vi "GUI_Single Button Pump.vi"() -> ()   [LabVIEW 2011] (continued)
                            n349 = call "MID-VAC Timer.vi"("TO sec (Start timer)"=30.0, "Action"=timerAction_typdef."Start Timer") -> ()  [unwired: 9 in, 1 out]
                            n350 = Concatenate Strings("Main: HPD Sanity Check>>", w961) -> (w960:string)
                          }
                          frame "Continue to Wait" {
                            # "Continue to wait. Reset Timer"
                            n351 = call "MID-VAC Timer.vi"("TO sec (Start timer)"=30.0, "Action"=timerAction_typdef."Start Timer") -> ()  [unwired: 9 in, 1 out]
                            n352 = Concatenate Strings("Main: HPD Sanity Check>>", w965) -> (w966:string)
                          }
                          frame "Exit" {
                          }
                        }
                      }
                      frame True {
                        n353 = Concatenate Strings("Main: HPD Sanity Check>>", w972) -> (w971:string)
                      }
                    }
                  }
                }
                n354 = call "MID-VAC Timer.vi"("Action"=timerAction_typdef."Timer Running") -> ("TO"=w925:bool)  [unwired: 10 in]
                n355 = And(x=w920, y=w925) -> (x .and. y?=w924:bool)
                n356 = Concatenate Strings(w916, " Valve is NOT Closed. Perform corrective action.\nClick on continue to wait for some more time.\nClick Exit to abort GPM" ("message")) -> (w917:string)
                n357 = call "Generate TO event.vi"("Boolean"=w924, "message"=w917, "User Event in"=w927) -> ()  [unwired: 9 in]
              }
            }
          }
        }
        n358 = call <vilib>:"Add State(s) to Queue__jki_lib_state_machine.vi"("State(s) in Front (\"\")"=w895, "State(s) in (\"\")"=w890) -> ("States Out"=w900:string)  [unwired: 13 in]
      }
      frame "Main: HPBD Sanity Check" {
        # "Check if gate valve between COMP and M123 is Open"
        n359 = Unbundle By Name(w976) -> ("Chamber Selection.M123"=w979:bool, "Chamber Selection.HPBD"=w980:bool)
        n360 = case shown="True" w980 {
          tunnel: w985 -> [w989 w998]
          tunnel: w984 -> [_ w997]
          tunnel: [w989 w996] -> w983
          tunnel: w982 -> [_ w995]
          tunnel: ["" w994] -> w981
          tunnel: w976 -> [w987 w993]
          tunnel: w979 -> [_ w991]
          tunnel: w978 -> [_ w992]
          tunnel: [w987 w990] -> w975
          frame False {
          }
          frame True {
            # "Check Conditions"
            n361 = case shown="\"False\", Default" w992 {
              selector: w992 -> [_ w1011]
              tunnel: w998 -> [w1003 w1013]
              tunnel: w997 -> [_ _]
              tunnel: [w1003 w1004] -> w996
              tunnel: w995 -> [_ _]
              tunnel: [w1001 ""] -> w994
              tunnel: w993 -> [w999 w1010]
              tunnel: w991 -> [w1000 _]
              tunnel: [w999 w1009] -> w990
              frame "False", Default {
                w1002 = "Main: HPBD Sanity Check>>M123-HPBD"
                # "COMP SELECTED?"
                n362 = Select(t=w1002, s=w1000, f=w1002) -> (s? t:f=w1001:string)
              }
              frame "M123-HPBD" {
                # "Event TAG"
                n363 = case shown="\"M123-HPBD\"" w1011 {
                  tunnel: [w1015 w1016] -> w1014
                  frame "False", Default {
                    w1015 = T32[] [enum."No Action"] items=["No Action", "Is EC GPM Mode ON?", "Is EC GPM Mode Off?", "Is EC GVM Mode ON?", "Is EC GVM Off?", "Is  EC GPM or GVM Mode ON?", "Is LB GPM Mode ON?", "Is LB GPM Mode Off?", "Is LB GVM Mode ON?", "Is LB GVM Mode Off?", "Is  LB GPM or GVM Mode ON?", "Is M123 Turbo Gate Valve Opened? ", "Is M123 Turbo Gate Valve Closed?", "Is OAP Turbo Gate Valve Opened?", "Is OAP Turbo Gate Valve Closed?", "Is BTLTurbo Gate Valve Opened?", "Is BTL Turbo Gate Valve Closed?", "Is TARGET Turbo Gate Valve 1Opened?", "Is TARGET1 Turbo Gate Valve Closed?", "Is TARGET Turbo Gate Valve 2 Opened?", "Is TAREGT2 Turbo Gate Valve Closed?", "Is BTL2 Turbo Gate Valve Opened?", "Is BTL2 Turbo Gate Valve Closed?", "Is HPD Turbo Gate Valve Opened?", "Is HPD Turbo Gate Valve Closed?", "Is COMP to M123 gate Valve Opened?", "Is COMP to M123 Valve Closed?", "Is HPBD Gate Valve Opened?", "Is HPBD Gate Valve Closed?", "Is M123 to OAP gate valve opened?", "Is M123 to OAP gate valve closed?", "Is OAP to BLT gate valve opened?", "Is OAP to BTL Gate Valve Closed?", "Is BLT to TARGET gate valve opened?", "Is BTL to TARGET Gate Valve Closed?", "Is TARGET to BLT2 gate valve opened?", "Is TARGET to BTL2 Gate Valve Closed?", "Is BLT2 to HPD gate valve opened?", "Is BTL2 to HPD Gate Valve Closed?", "Is COMP at Atmospheric Pressure?", "Is M123 at Atmospheric Pressure?", "Is BeamDump at Atmospheric Pressure?", "Is OAP at Atmospheric Pressure?", "Is BLT at Atmospheric Pressure", "Is TARGET at Atmospheric Pressure?", "Is BLT2 at Atmospheric Pressure?", "Is HPD at Atmospheric Pressure?", "Is the EC Roughing Pump ON?", "Is the EC Roughing Pump OFF?", "Does the EC Roughing Pump have a fault?", "Is the LB Roughing Pump ON?", "Is the LB Roughing Pump Off?", "Does the LB Roughing Pump have a fault?", "Is the EC Backing Pump ON?", "Is the EC Backing Pump OFF?", "Is the LB Backing Pump ON?", "Is the LB Backing Pump OFF?", "Does the EC Backing Pump have a fault?", "Does the LB Backing Pump have a fault?", "Is the EC Backing Pipe at Atmospheric Pressure", "Is the LB Backing Pipe at Atmospheric Pressure", "Is the EC Backing Manifold at Atmospheric Pressure", "s the LB Backing Manifold at Atmospheric Pressure?", "Is the EC Roughing Pipe at Atmospheric Pressure", "Is the LB Roughing Pipe at Atmospheric Pressure?", "Is the EC Roughing Manifold at Atmospheric Pressure", "Is the LB Roughing Manifold at Atmospheric Pressure", "Is LB Backing Manifold Valve Opened?", "Is EC Backing Manifold Valve Opened?", "Is LB Roughing Manifold Valve Opened?", "Is EC Roughing Manifold Valve Opened?", "Is COMP Roughing Valve Opened?", "Is M123 Roughing Valve Opened?", "Is M123 Roughing Valve Closed?", "Is OAP Roughing Valve Opened?", "Is OAP Roughing Valve Closed?", "Is HPBD Roughing Valve Opened?", "Is HPBD Roughing Valve Closed?", "Is BTL Roughing Valve Opened?", "Is BTL Roughing Valve Closed?", "Is TARGET Roughing Valve Opened?", "Is TARGET Roughing Valve Closed?", "Is BTL2 Roughing Valve Opened?", "Is BTL2 Roughing Valve Closed?", "Is HPD Roughing Valve Opened?", "Is HPD Roughing Valve Closed?", "Is COMP Turbo Backing Valve Opened?", "Is M123 Turbo Backing Valve Opened", "Is HPBD Turbo Backing Valve Opened?", "Is OAP Turbo Backing Valve Opened?", "Is BTL Turbo Backing Valve Opened?", "Is TARGET1 Turbo Backing Valve Opened?", "Is TARGET2 Turbo Backing Valve Opened?", "Is BTL2 Turbo Backing Valve Opened?", "Is HPD Turbo Backing Valve Opened?", "Is M123 Backing at MID-VAC?", "Is OAP Backing at MID-VAC?", "Is TARGET1 Backing at MID-VAC?", "Is TARGET2 Backing at MID-VAC?", "Is BTL Backing at MID-VAC?", "Is BTL2 Backing at MID-VAC?", "Is HPD Backing at MID-VAC?", "Is M123 Turbo in Normal Operation", "Is COMP Turbo in Normal Operation", "Is OAP Turbo in Normal Operation", "Is BTL Turbo in Normal Operation", "Is TARGET1 Turbo in Normal Operation", "Is TARGET2 Turbo in Normal Operation", "Is BTL2 Turbo in Normal Operation", "Is HPD Turbo in Normal Operation", "Is M123 at MID-VAC?", "Is OAP at MID-VAC?", "Is COMP at MID-VAC?", "Is BTL at MID-VAC?", "Is TARGET at MID-VAC?", "Is BTL2 at MID-VAC?", "Is HPD at MID-VAC?"]
                  }
                  frame "M123-HPBD" {
                    w1016 = T32[] [enum."Is HPBD Gate Valve Closed?"] items=["No Action", "Is EC GPM Mode ON?", "Is EC GPM Mode Off?", "Is EC GVM Mode ON?", "Is EC GVM Off?", "Is  EC GPM or GVM Mode ON?", "Is LB GPM Mode ON?", "Is LB GPM Mode Off?", "Is LB GVM Mode ON?", "Is LB GVM Mode Off?", "Is  LB GPM or GVM Mode ON?", "Is M123 Turbo Gate Valve Opened? ", "Is M123 Turbo Gate Valve Closed?", "Is OAP Turbo Gate Valve Opened?", "Is OAP Turbo Gate Valve Closed?", "Is BTLTurbo Gate Valve Opened?", "Is BTL Turbo Gate Valve Closed?", "Is TARGET Turbo Gate Valve 1Opened?", "Is TARGET1 Turbo Gate Valve Closed?", "Is TARGET Turbo Gate Valve 2 Opened?", "Is TAREGT2 Turbo Gate Valve Closed?", "Is BTL2 Turbo Gate Valve Opened?", "Is BTL2 Turbo Gate Valve Closed?", "Is HPD Turbo Gate Valve Opened?", "Is HPD Turbo Gate Valve Closed?", "Is COMP to M123 gate Valve Opened?", "Is COMP to M123 Valve Closed?", "Is HPBD Gate Valve Opened?", "Is HPBD Gate Valve Closed?", "Is M123 to OAP gate valve opened?", "Is M123 to OAP gate valve closed?", "Is OAP to BLT gate valve opened?", "Is OAP to BTL Gate Valve Closed?", "Is BLT to TARGET gate valve opened?", "Is BTL to TARGET Gate Valve Closed?", "Is TARGET to BLT2 gate valve opened?", "Is TARGET to BTL2 Gate Valve Closed?", "Is BLT2 to HPD gate valve opened?", "Is BTL2 to HPD Gate Valve Closed?", "Is COMP at Atmospheric Pressure?", "Is M123 at Atmospheric Pressure?", "Is BeamDump at Atmospheric Pressure?", "Is OAP at Atmospheric Pressure?", "Is BLT at Atmospheric Pressure", "Is TARGET at Atmospheric Pressure?", "Is BLT2 at Atmospheric Pressure?", "Is HPD at Atmospheric Pressure?", "Is the EC Roughing Pump ON?", "Is the EC Roughing Pump OFF?", "Does the EC Roughing Pump have a fault?", "Is the LB Roughing Pump ON?", "Is the LB Roughing Pump Off?", "Does the LB Roughing Pump have a fault?", "Is the EC Backing Pump ON?", "Is the EC Backing Pump OFF?", "Is the LB Backing Pump ON?", "Is the LB Backing Pump OFF?", "Does the EC Backing Pump have a fault?", "Does the LB Backing Pump have a fault?", "Is the EC Backing Pipe at Atmospheric Pressure", "Is the LB Backing Pipe at Atmospheric Pressure", "Is the EC Backing Manifold at Atmospheric Pressure", "s the LB Backing Manifold at Atmospheric Pressure?", "Is the EC Roughing Pipe at Atmospheric Pressure", "Is the LB Roughing Pipe at Atmospheric Pressure?", "Is the EC Roughing Manifold at Atmospheric Pressure", "Is the LB Roughing Manifold at Atmospheric Pressure", "Is LB Backing Manifold Valve Opened?", "Is EC Backing Manifold Valve Opened?", "Is LB Roughing Manifold Valve Opened?", "Is EC Roughing Manifold Valve Opened?", "Is COMP Roughing Valve Opened?", "Is M123 Roughing Valve Opened?", "Is M123 Roughing Valve Closed?", "Is OAP Roughing Valve Opened?", "Is OAP Roughing Valve Closed?", "Is HPBD Roughing Valve Opened?", "Is HPBD Roughing Valve Closed?", "Is BTL Roughing Valve Opened?", "Is BTL Roughing Valve Closed?", "Is TARGET Roughing Valve Opened?", "Is TARGET Roughing Valve Closed?", "Is BTL2 Roughing Valve Opened?", "Is BTL2 Roughing Valve Closed?", "Is HPD Roughing Valve Opened?", "Is HPD Roughing Valve Closed?", "Is COMP Turbo Backing Valve Opened?", "Is M123 Turbo Backing Valve Opened", "Is HPBD Turbo Backing Valve Opened?", "Is OAP Turbo Backing Valve Opened?", "Is BTL Turbo Backing Valve Opened?", "Is TARGET1 Turbo Backing Valve Opened?", "Is TARGET2 Turbo Backing Valve Opened?", "Is BTL2 Turbo Backing Valve Opened?", "Is HPD Turbo Backing Valve Opened?", "Is M123 Backing at MID-VAC?", "Is OAP Backing at MID-VAC?", "Is TARGET1 Backing at MID-VAC?", "Is TARGET2 Backing at MID-VAC?", "Is BTL Backing at MID-VAC?", "Is BTL2 Backing at MID-VAC?", "Is HPD Backing at MID-VAC?", "Is M123 Turbo in Normal Operation", "Is COMP Turbo in Normal Operation", "Is OAP Turbo in Normal Operation", "Is BTL Turbo in Normal Operation", "Is TARGET1 Turbo in Normal Operation", "Is TARGET2 Turbo in Normal Operation", "Is BTL2 Turbo in Normal Operation", "Is HPD Turbo in Normal Operation", "Is M123 at MID-VAC?", "Is OAP at MID-VAC?", "Is COMP at MID-VAC?", "Is BTL at MID-VAC?", "Is TARGET at MID-VAC?", "Is BTL2 at MID-VAC?", "Is HPD at MID-VAC?"]
                  }
                }
                n364 = call "GetAction.vi"("Check Condition"=Error_codes."999-No Event" ("Error Codes"), "Query Array"=w1014, "error in (no error)"=w1013) -> ("Results Array"=w1007:bool[], "error out"=w1004:errorcluster)  [unwired: 7 in, 4 out]
                n365 = Index Array(array=w1007, index=0) -> (element=w1005:bool)
                n366 = Bundle By Name(cluster=w1010, "Isolate HPBD"=w1005) -> (w1009:T20)
              }
            }
          }
        }
        n367 = call <vilib>:"Add State(s) to Queue__jki_lib_state_machine.vi"("State(s) in Front (\"\")"=w981, "State(s) in (\"\")"=w977) -> ("States Out"=w986:string)  [unwired: 13 in]
      }
      frame "Main: Check COMP gate valve" {
        w1028 = Error_codes."003-Chamber Gate Valve Status" ("Error Codes")
        w1034 = T32[] [enum."Is COMP to M123 Valve Closed?"] items=["No Action", "Is EC GPM Mode ON?", "Is EC GPM Mode Off?", "Is EC GVM Mode ON?", "Is EC GVM Off?", "Is  EC GPM or GVM Mode ON?", "Is LB GPM Mode ON?", "Is LB GPM Mode Off?", "Is LB GVM Mode ON?", "Is LB GVM Mode Off?", "Is  LB GPM or GVM Mode ON?", "Is M123 Turbo Gate Valve Opened? ", "Is M123 Turbo Gate Valve Closed?", "Is OAP Turbo Gate Valve Opened?", "Is OAP Turbo Gate Valve Closed?", "Is BTLTurbo Gate Valve Opened?", "Is BTL Turbo Gate Valve Closed?", "Is TARGET Turbo Gate Valve 1Opened?", "Is TARGET1 Turbo Gate Valve Closed?", "Is TARGET Turbo Gate Valve 2 Opened?", "Is TAREGT2 Turbo Gate Valve Closed?", "Is BTL2 Turbo Gate Valve Opened?", "Is BTL2 Turbo Gate Valve Closed?", "Is HPD Turbo Gate Valve Opened?", "Is HPD Turbo Gate Valve Closed?", "Is COMP to M123 gate Valve Opened?", "Is COMP to M123 Valve Closed?", "Is HPBD Gate Valve Opened?", "Is HPBD Gate Valve Closed?", "Is M123 to OAP gate valve opened?", "Is M123 to OAP gate valve closed?", "Is OAP to BLT gate valve opened?", "Is OAP to BTL Gate Valve Closed?", "Is BLT to TARGET gate valve opened?", "Is BTL to TARGET Gate Valve Closed?", "Is TARGET to BLT2 gate valve opened?", "Is TARGET to BTL2 Gate Valve Closed?", "Is BLT2 to HPD gate valve opened?", "Is BTL2 to HPD Gate Valve Closed?", "Is COMP at Atmospheric Pressure?", "Is M123 at Atmospheric Pressure?", "Is BeamDump at Atmospheric Pressure?", "Is OAP at Atmospheric Pressure?", "Is BLT at Atmospheric Pressure", "Is TARGET at Atmospheric Pressure?", "Is BLT2 at Atmospheric Pressure?", "Is HPD at Atmospheric Pressure?", "Is the EC Roughing Pump ON?", "Is the EC Roughing Pump OFF?", "Does the EC Roughing Pump have a fault?", "Is the LB Roughing Pump ON?", "Is the LB Roughing Pump Off?", "Does the LB Roughing Pump have a fault?", "Is the EC Backing Pump ON?", "Is the EC Backing Pump OFF?", "Is the LB Backing Pump ON?", "Is the LB Backing Pump OFF?", "Does the EC Backing Pump have a fault?", "Does the LB Backing Pump have a fault?", "Is the EC Backing Pipe at Atmospheric Pressure", "Is the LB Backing Pipe at Atmospheric Pressure", "Is the EC Backing Manifold at Atmospheric Pressure", "s the LB Backing Manifold at Atmospheric Pressure?", "Is the EC Roughing Pipe at Atmospheric Pressure", "Is the LB Roughing Pipe at Atmospheric Pressure?", "Is the EC Roughing Manifold at Atmospheric Pressure", "Is the LB Roughing Manifold at Atmospheric Pressure", "Is LB Backing Manifold Valve Opened?", "Is EC Backing Manifold Valve Opened?", "Is LB Roughing Manifold Valve Opened?", "Is EC Roughing Manifold Valve Opened?", "Is COMP Roughing Valve Opened?", "Is M123 Roughing Valve Opened?", "Is M123 Roughing Valve Closed?", "Is OAP Roughing Valve Opened?", "Is OAP Roughing Valve Closed?", "Is HPBD Roughing Valve Opened?", "Is HPBD Roughing Valve Closed?", "Is BTL Roughing Valve Opened?", "Is BTL Roughing Valve Closed?", "Is TARGET Roughing Valve Opened?", "Is TARGET Roughing Valve Closed?", "Is BTL2 Roughing Valve Opened?", "Is BTL2 Roughing Valve Closed?", "Is HPD Roughing Valve Opened?", "Is HPD Roughing Valve Closed?", "Is COMP Turbo Backing Valve Opened?", "Is M123 Turbo Backing Valve Opened", "Is HPBD Turbo Backing Valve Opened?", "Is OAP Turbo Backing Valve Opened?", "Is BTL Turbo Backing Valve Opened?", "Is TARGET1 Turbo Backing Valve Opened?", "Is TARGET2 Turbo Backing Valve Opened?", "Is BTL2 Turbo Backing Valve Opened?", "Is HPD Turbo Backing Valve Opened?", "Is M123 Backing at MID-VAC?", "Is OAP Backing at MID-VAC?", "Is TARGET1 Backing at MID-VAC?", "Is TARGET2 Backing at MID-VAC?", "Is BTL Backing at MID-VAC?", "Is BTL2 Backing at MID-VAC?", "Is HPD Backing at MID-VAC?", "Is M123 Turbo in Normal Operation", "Is COMP Turbo in Normal Operation", "Is OAP Turbo in Normal Operation", "Is BTL Turbo in Normal Operation", "Is TARGET1 Turbo in Normal Operation", "Is TARGET2 Turbo in Normal Operation", "Is BTL2 Turbo in Normal Operation", "Is HPD Turbo in Normal Operation", "Is M123 at MID-VAC?", "Is OAP at MID-VAC?", "Is COMP at MID-VAC?", "Is BTL at MID-VAC?", "Is TARGET at MID-VAC?", "Is BTL2 at MID-VAC?", "Is HPD at MID-VAC?"]
        # "Event TAG"
        # "Check Conditions"
        # "Check if gate valve between COMP and M123 is Open"
        n368 = call "GetAction.vi"("Check Condition"=w1028, "Query Array"=w1034, "error in (no error)"=w1033) -> ("Status Array Out"=w1029:string[], "Generate Event?"=w1021:bool, "error out"=w1031:errorcluster)  [unwired: 7 in, 3 out]
        n369 = Unbundle By Name(w1025) -> ("VI Refnum"=w1024:refnum<vi>)
        n370 = call "Generate User Event.vi"("Add(t)/Remove(f) Event"=w1021, "error in (no error)"=w1031, "User Event in"=w1032, "Status Array In"=w1029, "Error Codes"=w1028) -> ("error out"=w1030:errorcluster)  [unwired: 5 in, 1 out]
        n371 = Not A Number/Path/Refnum?(number/path/refnum=w1024) -> (NaN/Path/Refnum?=w1023:bool)
        n372 = call "MID-VAC Timer.vi"("Action"=timerAction_typdef."Timer Running") -> ("TO"=w1026:bool)  [unwired: 10 in]
        n373 = case shown="False" w1021 {
          tunnel: ["Main: Check Chamber Pressure" w1050] -> w1022
          tunnel: w1024 -> [w1040 w1049]
          tunnel: w1023 -> [w1041 w1048]
          frame False {
            n374 = case shown="True" w1041 {
              tunnel: w1040 -> [_ w1044]
              frame False {
              }
              frame True {
                n375 = invoke class="VI" method="Abort VI"(reference=w1044) -> (reference out=w1042:refnum<vi>, error out=w1043:errorcluster)  [unwired: 2 in, 1 out]
                n376 = case shown="No Error" w1043 {
                  selector: w1043 -> [w1046 _]
                  tunnel: w1042 -> [w1047 _]
                  frame No Error {
                    n377 = Close Reference(reference=w1047, error in (no error)=w1046) -> (error out=w1045:errorcluster)
                    n378 = invoke on="User Input Panel" class="SubPnl" method="Remove VI"(error in=w1045) -> ()  [unwired: 2 in, 3 out]
                  }
                  frame Error {
                  }
                }
              }
            }
            n379 = call "MID-VAC Timer.vi"("TO sec (Start timer)"=1.0, "Action"=timerAction_typdef."Start Timer") -> ()  [unwired: 9 in, 1 out]
          }
          frame True {
            # "when to is true\nand"
            n380 = case shown="False" w1048 {
              tunnel: w1049 -> [w1054 _]
              tunnel: [w1052 "Main: Check COMP gate valve"] -> w1050
              frame False {
                n381 = call "FindControlByName_VEPS.vi"("control name"="Op Out", "vi refnum"=w1054) -> ("control refnum"=w1056:refnum<vi>)  [unwired: 2 in, 1 out]
                n382 = property class="Ctl"(reference=w1056) -> ("Value"=w1055:variant)  [unwired: 1 in, 2 out]
                n383 = Variant To Data(type=op_typdef."Idle" ("Op Out"), Variant=w1055) -> (data=w1053:T24)  [unwired: 1 in, 1 out]
                n384 = case shown="\"Idle\", Default" w1053 {
                  tunnel: ["Main: Check COMP gate valve" "Main: Check COMP gate valve" "Idle\nMacro: Exit"] -> w1052
                  frame "Idle", Default {
                    n385 = call "MID-VAC Timer.vi"("TO sec (Start timer)"=30.0, "Action"=timerAction_typdef."Start Timer") -> ()  [unwired: 9 in, 1 out]
                  }
                  frame "Continue to Wait" {
                    # "Continue to wait. Reset Timer"
                    n386 = call "MID-VAC Timer.vi"("TO sec (Start timer)"=30.0, "Action"=timerAction_typdef."Start Timer") -> ()  [unwired: 9 in, 1 out]
                  }
                  frame "Exit" {
                  }
                }
              }
              frame True {
              }
            }
          }
        }
        n387 = And(x=w1021, y=w1026) -> (x .and. y?=w1018:bool)
        n388 = call "Generate TO event.vi"("Boolean"=w1018, "message"="The COMP to M123 Valve is NOT Closed.\nClick on continue to wait for some more time.\nClick Exit to abort GPM", "User Event in"=w1020) -> ()  [unwired: 9 in]
        n389 = call <vilib>:"Add State(s) to Queue__jki_lib_state_machine.vi"("State(s) in Front (\"\")"=w1022, "State(s) in (\"\")"=w1036) -> ("States Out"=w1035:string)  [unwired: 13 in]
      }
      frame "Main: Check Chamber Pressure" {
        w1073 = Error_codes."004-Check Chamber Pressures" ("Error Codes")
        w1092 = T32[] [enum."Is HPBD Gate Valve Opened?"] items=["No Action", "Is EC GPM Mode ON?", "Is EC GPM Mode Off?", "Is EC GVM Mode ON?", "Is EC GVM Off?", "Is  EC GPM or GVM Mode ON?", "Is LB GPM Mode ON?", "Is LB GPM Mode Off?", "Is LB GVM Mode ON?", "Is LB GVM Mode Off?", "Is  LB GPM or GVM Mode ON?", "Is M123 Turbo Gate Valve Opened? ", "Is M123 Turbo Gate Valve Closed?", "Is OAP Turbo Gate Valve Opened?", "Is OAP Turbo Gate Valve Closed?", "Is BTLTurbo Gate Valve Opened?", "Is BTL Turbo Gate Valve Closed?", "Is TARGET Turbo Gate Valve 1Opened?", "Is TARGET1 Turbo Gate Valve Closed?", "Is TARGET Turbo Gate Valve 2 Opened?", "Is TAREGT2 Turbo Gate Valve Closed?", "Is BTL2 Turbo Gate Valve Opened?", "Is BTL2 Turbo Gate Valve Closed?", "Is HPD Turbo Gate Valve Opened?", "Is HPD Turbo Gate Valve Closed?", "Is COMP to M123 gate Valve Opened?", "Is COMP to M123 Valve Closed?", "Is HPBD Gate Valve Opened?", "Is HPBD Gate Valve Closed?", "Is M123 to OAP gate valve opened?", "Is M123 to OAP gate valve closed?", "Is OAP to BLT gate valve opened?", "Is OAP to BTL Gate Valve Closed?", "Is BLT to TARGET gate valve opened?", "Is BTL to TARGET Gate Valve Closed?", "Is TARGET to BLT2 gate valve opened?", "Is TARGET to BTL2 Gate Valve Closed?", "Is BLT2 to HPD gate valve opened?", "Is BTL2 to HPD Gate Valve Closed?", "Is COMP at Atmospheric Pressure?", "Is M123 at Atmospheric Pressure?", "Is BeamDump at Atmospheric Pressure?", "Is OAP at Atmospheric Pressure?", "Is BLT at Atmospheric Pressure", "Is TARGET at Atmospheric Pressure?", "Is BLT2 at Atmospheric Pressure?", "Is HPD at Atmospheric Pressure?", "Is the EC Roughing Pump ON?", "Is the EC Roughing Pump OFF?", "Does the EC Roughing Pump have a fault?", "Is the LB Roughing Pump ON?", "Is the LB Roughing Pump Off?", "Does the LB Roughing Pump have a fault?", "Is the EC Backing Pump ON?", "Is the EC Backing Pump OFF?", "Is the LB Backing Pump ON?", "Is the LB Backing Pump OFF?", "Does the EC Backing Pump have a fault?", "Does the LB Backing Pump have a fault?", "Is the EC Backing Pipe at Atmospheric Pressure", "Is the LB Backing Pipe at Atmospheric Pressure", "Is the EC Backing Manifold at Atmospheric Pressure", "s the LB Backing Manifold at Atmospheric Pressure?", "Is the EC Roughing Pipe at Atmospheric Pressure", "Is the LB Roughing Pipe at Atmospheric Pressure?", "Is the EC Roughing Manifold at Atmospheric Pressure", "Is the LB Roughing Manifold at Atmospheric Pressure", "Is LB Backing Manifold Valve Opened?", "Is EC Backing Manifold Valve Opened?", "Is LB Roughing Manifold Valve Opened?", "Is EC Roughing Manifold Valve Opened?", "Is COMP Roughing Valve Opened?", "Is M123 Roughing Valve Opened?", "Is M123 Roughing Valve Closed?", "Is OAP Roughing Valve Opened?", "Is OAP Roughing Valve Closed?", "Is HPBD Roughing Valve Opened?", "Is HPBD Roughing Valve Closed?", "Is BTL Roughing Valve Opened?", "Is BTL Roughing Valve Closed?", "Is TARGET Roughing Valve Opened?", "Is TARGET Roughing Valve Closed?", "Is BTL2 Roughing Valve Opened?", "Is BTL2 Roughing Valve Closed?", "Is HPD Roughing Valve Opened?", "Is HPD Roughing Valve Closed?", "Is COMP Turbo Backing Valve Opened?", "Is M123 Turbo Backing Valve Opened", "Is HPBD Turbo Backing Valve Opened?", "Is OAP Turbo Backing Valve Opened?", "Is BTL Turbo Backing Valve Opened?", "Is TARGET1 Turbo Backing Valve Opened?", "Is TARGET2 Turbo Backing Valve Opened?", "Is BTL2 Turbo Backing Valve Opened?", "Is HPD Turbo Backing Valve Opened?", "Is M123 Backing at MID-VAC?", "Is OAP Backing at MID-VAC?", "Is TARGET1 Backing at MID-VAC?", "Is TARGET2 Backing at MID-VAC?", "Is BTL Backing at MID-VAC?", "Is BTL2 Backing at MID-VAC?", "Is HPD Backing at MID-VAC?", "Is M123 Turbo in Normal Operation", "Is COMP Turbo in Normal Operation", "Is OAP Turbo in Normal Operation", "Is BTL Turbo in Normal Operation", "Is TARGET1 Turbo in Normal Operation", "Is TARGET2 Turbo in Normal Operation", "Is BTL2 Turbo in Normal Operation", "Is HPD Turbo in Normal Operation", "Is M123 at MID-VAC?", "Is OAP at MID-VAC?", "Is COMP at MID-VAC?", "Is BTL at MID-VAC?", "Is TARGET at MID-VAC?", "Is BTL2 at MID-VAC?", "Is HPD at MID-VAC?"]
        # "If F, then all chambers are at ATM"
        # "Check Conditions"
        # "Check if Any Chamber is NOT at ATM?"
        n390 = call "GetAction.vi"("Check Condition"=Error_codes."999-No Event" ("Error Codes"), "Query Array"=w1092, "error in (no error)"=w1091) -> ("Results Array"=w1086:bool[], "error out"=w1089:errorcluster)  [unwired: 7 in, 4 out]
        n391 = Index Array(array=w1086, index=0) -> (element=w1072:bool)
        n392 = Not(x=w1072) -> (.not. x?=w1067:bool)
        n393 = Unbundle By Name(w1071) -> ("Chamber Selection"=w1070:T21)
        n394 = call "Selection ActionBuilder.vi"("Selection Action"=Selection_Action_typdef."Check Chamber Pressure", "Isolate HPBD"=w1067, "Chamber Selection"=w1070) -> ("Action Array Out"=w1068:T32[])  [unwired: 7 in, 1 out]
        n395 = call "GetAction.vi"("Check Condition"=w1073, "Query Array"=w1068, "input cluster"=w1071, "error in (no error)"=w1089) -> ("Status Array Out"=w1075:string[], "Generate Event?"=w1080:bool, "error out"=w1074:errorcluster)  [unwired: 6 in, 3 out]
        n396 = call "Generate User Event.vi"("Add(t)/Remove(f) Event"=w1080, "error in (no error)"=w1074, "User Event in"=w1090, "Status Array In"=w1075, "Error Codes"=w1073) -> ("error out"=w1088:errorcluster)  [unwired: 5 in, 1 out]
        n397 = Unbundle By Name(w1071) -> ("VI Refnum"=w1082:refnum<vi>)
        n398 = Not A Number/Path/Refnum?(number/path/refnum=w1082) -> (NaN/Path/Refnum?=w1081:bool)
        n399 = Bundle By Name(cluster=w1071, "Isolate HPBD"=w1067) -> (w1087:T20)
        n400 = case shown="False" w1080 {
          tunnel: ["Main: Check GPM GVM Mode Status" w1109] -> w1079
          tunnel: w1082 -> [w1099 w1108]
          tunnel: w1081 -> [w1100 w1107]
          frame False {
            n401 = case shown="True" w1100 {
              tunnel: w1099 -> [_ w1103]
              frame False {
              }
              frame True {
                n402 = invoke class="VI" method="Abort VI"(reference=w1103) -> (reference out=w1101:refnum<vi>, error out=w1102:errorcluster)  [unwired: 2 in, 1 out]
                n403 = case shown="No Error" w1102 {
                  selector: w1102 -> [w1105 _]
                  tunnel: w1101 -> [w1106 _]
                  frame No Error {
                    n404 = Close Reference(reference=w1106, error in (no error)=w1105) -> (error out=w1104:errorcluster)
                    n405 = invoke on="User Input Panel" class="SubPnl" method="Remove VI"(error in=w1104) -> ()  [unwired: 2 in, 3 out]
                  }
                  frame Error {
                  }
                }
              }
            }
            n406 = call "MID-VAC Timer.vi"("TO sec (Start timer)"=1.0, "Action"=timerAction_typdef."Start Timer") -> ()  [unwired: 9 in, 1 out]
          }
          frame True {
            # "when to is true\nand"
            n407 = case shown="True" w1107 {
              tunnel: w1108 -> [w1113 _]
              tunnel: [w1111 "Main: Check Chamber Pressure"] -> w1109
              frame False {
                n408 = call "FindControlByName_VEPS.vi"("control name"="Op Out", "vi refnum"=w1113) -> ("control refnum"=w1115:refnum<vi>)  [unwired: 2 in, 1 out]
                n409 = property class="Ctl"(reference=w1115) -> ("Value"=w1114:variant)  [unwired: 1 in, 2 out]
                n410 = Variant To Data(type=op_typdef."Idle" ("Op Out"), Variant=w1114) -> (data=w1112:T24)  [unwired: 1 in, 1 out]
                n411 = case shown="\"Idle\", Default" w1112 {
                  tunnel: ["Main: Check Chamber Pressure" "Main: Check Chamber Pressure" "Idle\nMacro: Exit"] -> w1111
                  frame "Idle", Default {
                    n412 = call "MID-VAC Timer.vi"("TO sec (Start timer)"=30.0, "Action"=timerAction_typdef."Start Timer") -> ()  [unwired: 9 in, 1 out]
                  }
                  frame "Continue to Wait" {
                    # "Continue to wait. Reset Timer"
                    n413 = call "MID-VAC Timer.vi"("TO sec (Start timer)"=30.0, "Action"=timerAction_typdef."Start Timer") -> ()  [unwired: 9 in, 1 out]
                  }
                  frame "Exit" {
                  }
                }
              }
              frame True {
              }
            }
          }
        }
        n414 = call "MID-VAC Timer.vi"("Action"=timerAction_typdef."Timer Running") -> ("TO"=w1083:bool)  [unwired: 10 in]
        n415 = And(x=w1080, y=w1083) -> (x .and. y?=w1077:bool)
        n416 = call <vilib>:"Add State(s) to Queue__jki_lib_state_machine.vi"("State(s) in (\"\")"=w1095, "State(s) at Back (\"\")"=w1079) -> ("States Out"=w1094:string)  [unwired: 13 in]
        n417 = call "Generate TO event.vi"("Boolean"=w1077, "message"="Some of the chambers are not at Atmosphere. Entering GPM Mode is NOT allowed.\nPlease Vent chambers and proceed.\nClick on Exit to QUIT", "User Event in"=w1078) -> ()  [unwired: 9 in]
      }
      frame "Main: Check GPM GVM Mode Status" {
        w1134 = T32[] [enum."Is EC GPM Mode Off?", enum."Is LB GPM Mode Off?", enum."Is EC GVM Off?", enum."Is LB GVM Mode Off?"] items=["No Action", "Is EC GPM Mode ON?", "Is EC GPM Mode Off?", "Is EC GVM Mode ON?", "Is EC GVM Off?", "Is  EC GPM or GVM Mode ON?", "Is LB GPM Mode ON?", "Is LB GPM Mode Off?", "Is LB GVM Mode ON?", "Is LB GVM Mode Off?", "Is  LB GPM or GVM Mode ON?", "Is M123 Turbo Gate Valve Opened? ", "Is M123 Turbo Gate Valve Closed?", "Is OAP Turbo Gate Valve Opened?", "Is OAP Turbo Gate Valve Closed?", "Is BTLTurbo Gate Valve Opened?", "Is BTL Turbo Gate Valve Closed?", "Is TARGET Turbo Gate Valve 1Opened?", "Is TARGET1 Turbo Gate Valve Closed?", "Is TARGET Turbo Gate Valve 2 Opened?", "Is TAREGT2 Turbo Gate Valve Closed?", "Is BTL2 Turbo Gate Valve Opened?", "Is BTL2 Turbo Gate Valve Closed?", "Is HPD Turbo Gate Valve Opened?", "Is HPD Turbo Gate Valve Closed?", "Is COMP to M123 gate Valve Opened?", "Is COMP to M123 Valve Closed?", "Is HPBD Gate Valve Opened?", "Is HPBD Gate Valve Closed?", "Is M123 to OAP gate valve opened?", "Is M123 to OAP gate valve closed?", "Is OAP to BLT gate valve opened?", "Is OAP to BTL Gate Valve Closed?", "Is BLT to TARGET gate valve opened?", "Is BTL to TARGET Gate Valve Closed?", "Is TARGET to BLT2 gate valve opened?", "Is TARGET to BTL2 Gate Valve Closed?", "Is BLT2 to HPD gate valve opened?", "Is BTL2 to HPD Gate Valve Closed?", "Is COMP at Atmospheric Pressure?", "Is M123 at Atmospheric Pressure?", "Is BeamDump at Atmospheric Pressure?", "Is OAP at Atmospheric Pressure?", "Is BLT at Atmospheric Pressure", "Is TARGET at Atmospheric Pressure?", "Is BLT2 at Atmospheric Pressure?", "Is HPD at Atmospheric Pressure?", "Is the EC Roughing Pump ON?", "Is the EC Roughing Pump OFF?", "Does the EC Roughing Pump have a fault?", "Is the LB Roughing Pump ON?", "Is the LB Roughing Pump Off?", "Does the LB Roughing Pump have a fault?", "Is the EC Backing Pump ON?", "Is the EC Backing Pump OFF?", "Is the LB Backing Pump ON?", "Is the LB Backing Pump OFF?", "Does the EC Backing Pump have a fault?", "Does the LB Backing Pump have a fault?", "Is the EC Backing Pipe at Atmospheric Pressure", "Is the LB Backing Pipe at Atmospheric Pressure", "Is the EC Backing Manifold at Atmospheric Pressure", "s the LB Backing Manifold at Atmospheric Pressure?", "Is the EC Roughing Pipe at Atmospheric Pressure", "Is the LB Roughing Pipe at Atmospheric Pressure?", "Is the EC Roughing Manifold at Atmospheric Pressure", "Is the LB Roughing Manifold at Atmospheric Pressure", "Is LB Backing Manifold Valve Opened?", "Is EC Backing Manifold Valve Opened?", "Is LB Roughing Manifold Valve Opened?", "Is EC Roughing Manifold Valve Opened?", "Is COMP Roughing Valve Opened?", "Is M123 Roughing Valve Opened?", "Is M123 Roughing Valve Closed?", "Is OAP Roughing Valve Opened?", "Is OAP Roughing Valve Closed?", "Is HPBD Roughing Valve Opened?", "Is HPBD Roughing Valve Closed?", "Is BTL Roughing Valve Opened?", "Is BTL Roughing Valve Closed?", "Is TARGET Roughing Valve Opened?", "Is TARGET Roughing Valve Closed?", "Is BTL2 Roughing Valve Opened?", "Is BTL2 Roughing Valve Closed?", "Is HPD Roughing Valve Opened?", "Is HPD Roughing Valve Closed?", "Is COMP Turbo Backing Valve Opened?", "Is M123 Turbo Backing Valve Opened", "Is HPBD Turbo Backing Valve Opened?", "Is OAP Turbo Backing Valve Opened?", "Is BTL Turbo Backing Valve Opened?", "Is TARGET1 Turbo Backing Valve Opened?", "Is TARGET2 Turbo Backing Valve Opened?", "Is BTL2 Turbo Backing Valve Opened?", "Is HPD Turbo Backing Valve Opened?", "Is M123 Backing at MID-VAC?", "Is OAP Backing at MID-VAC?", "Is TARGET1 Backing at MID-VAC?", "Is TARGET2 Backing at MID-VAC?", "Is BTL Backing at MID-VAC?", "Is BTL2 Backing at MID-VAC?", "Is HPD Backing at MID-VAC?", "Is M123 Turbo in Normal Operation", "Is COMP Turbo in Normal Operation", "Is OAP Turbo in Normal Operation", "Is BTL Turbo in Normal Operation", "Is TARGET1 Turbo in Normal Operation", "Is TARGET2 Turbo in Normal Operation", "Is BTL2 Turbo in Normal Operation", "Is HPD Turbo in Normal Operation", "Is M123 at MID-VAC?", "Is OAP at MID-VAC?", "Is COMP at MID-VAC?", "Is BTL at MID-VAC?", "Is TARGET at MID-VAC?", "Is BTL2 at MID-VAC?", "Is HPD at MID-VAC?"]
        w1139 = Error_codes."001-GPM and GVM conditions" ("Error Codes")
        # "If F, then all chambers are at ATM"
        # "Event TAG"
        # "IS GPM or GVM Mode for EC and LB ON?"
        n418 = call "GetAction.vi"("Check Condition"=w1139, "Query Array"=w1134, "input cluster"=w1127, "error in (no error)"=w1141) -> ("Status Array Out"=w1140:string[], "Generate Event?"=w1128:bool, "error out"=w1137:errorcluster)  [unwired: 6 in, 3 out]
        n419 = case shown="\"PreCheck\"" w1135 {
          selector: w1135 -> [w1145 w1148 w1190]
          tunnel: [w1144 w1147 w1188] -> w1126
          tunnel: w1128 -> [_ _ _]
          tunnel: w1128 -> [_ w1152 w1189]
          tunnel: w1127 -> [_ w1151 w1191]
          frame "False", Default {
            # "Quit Option?"
            n420 = Concatenate Strings("Main: Check GPM GVM Mode Status>>", w1145) -> (w1144:string)
          }
          frame "PreCheck" {
            n421 = Unbundle By Name(w1151) -> ("VI Refnum"=w1149:refnum<vi>)
            n422 = Not A Number/Path/Refnum?(number/path/refnum=w1149) -> (NaN/Path/Refnum?=w1150:bool)
            n423 = case shown="False" w1152 {
              tunnel: ["Main: Check Turbo Gate Valves" w1167] -> w1147
              tunnel: w1149 -> [w1156 w1166]
              tunnel: w1150 -> [w1157 w1165]
              tunnel: w1148 -> [_ w1164]
              frame False {
                n424 = case shown="True" w1157 {
                  tunnel: w1156 -> [_ w1160]
                  frame False {
                  }
                  frame True {
                    n425 = invoke class="VI" method="Abort VI"(reference=w1160) -> (reference out=w1158:refnum<vi>, error out=w1159:errorcluster)  [unwired: 2 in, 1 out]
                    n426 = case shown="No Error" w1159 {
                      selector: w1159 -> [w1162 _]
                      tunnel: w1158 -> [w1163 _]
                      frame No Error {
                        n427 = Close Reference(reference=w1163, error in (no error)=w1162) -> (error out=w1161:errorcluster)
                        n428 = invoke on="User Input Panel" class="SubPnl" method="Remove VI"(error in=w1161) -> ()  [unwired: 2 in, 3 out]
                      }
                      frame Error {
                      }
                    }
                  }
                }
                n429 = call "MID-VAC Timer.vi"("TO sec (Start timer)"=1.0, "Action"=timerAction_typdef."Start Timer") -> ()  [unwired: 9 in, 1 out]
              }
              frame True {
                # "when to is true\nand"
                n430 = case shown="False" w1165 {
                  tunnel: w1166 -> [w1172 _]
                  tunnel: [w1170 w1185] -> w1167
                  tunnel: w1164 -> [w1168 w1186]
                  frame False {
                    n431 = call "FindControlByName_VEPS.vi"("control name"="Op Out", "vi refnum"=w1172) -> ("control refnum"=w1174:refnum<vi>)  [unwired: 2 in, 1 out]
                    n432 = property class="Ctl"(reference=w1174) -> ("Value"=w1173:variant)  [unwired: 1 in, 2 out]
                    n433 = Variant To Data(type=op_typdef."Idle" ("Op Out"), Variant=w1173) -> (data=w1171:T24)  [unwired: 1 in, 1 out]
                    n434 = case shown="\"Idle\", Default" w1171 {
                      tunnel: [w1176 "Main: Check Chamber Pressure" "Idle\nMacro: Exit"] -> w1170
                      tunnel: w1168 -> [w1177 _ _]
                      frame "Idle", Default {
                        n435 = call "MID-VAC Timer.vi"("TO sec (Start timer)"=30.0, "Action"=timerAction_typdef."Start Timer") -> ()  [unwired: 9 in, 1 out]
                        n436 = Concatenate Strings("Main: Check GPM GVM Mode Status>>", w1177) -> (w1176:string)
                      }
                      frame "Continue to Wait" {
                        # "Continue to wait. Reset Timer"
                        n437 = call "MID-VAC Timer.vi"("TO sec (Start timer)"=30.0, "Action"=timerAction_typdef."Start Timer") -> ()  [unwired: 9 in, 1 out]
                      }
                      frame "Exit" {
                      }
                    }
                  }
                  frame True {
                    n438 = Concatenate Strings("Main: Check GPM GVM Mode Status>>", w1186) -> (w1185:string)
                  }
                }
              }
            }
          }
          frame "end" {
            n439 = Unbundle By Name(w1191) -> ("VI Refnum"=w1192:refnum<vi>)
            n440 = Not A Number/Path/Refnum?(number/path/refnum=w1192) -> (NaN/Path/Refnum?=w1193:bool)
            n441 = case shown="False" w1189 {
              tunnel: ["Main: Open Turbo Gate Valves" w1208] -> w1188
              tunnel: w1192 -> [w1197 w1207]
              tunnel: w1193 -> [w1198 w1206]
              tunnel: w1190 -> [_ w1205]
              frame False {
                n442 = case shown="True" w1198 {
                  tunnel: w1197 -> [_ w1201]
                  frame False {
                  }
                  frame True {
                    n443 = invoke class="VI" method="Abort VI"(reference=w1201) -> (reference out=w1199:refnum<vi>, error out=w1200:errorcluster)  [unwired: 2 in, 1 out]
                    n444 = case shown="No Error" w1200 {
                      selector: w1200 -> [w1203 _]
                      tunnel: w1199 -> [w1204 _]
                      frame No Error {
                        n445 = Close Reference(reference=w1204, error in (no error)=w1203) -> (error out=w1202:errorcluster)
                        n446 = invoke on="User Input Panel" class="SubPnl" method="Remove VI"(error in=w1202) -> ()  [unwired: 2 in, 3 out]
                      }
                      frame Error {
                      }
                    }
                  }
                }
                n447 = call "MID-VAC Timer.vi"("TO sec (Start timer)"=1.0, "Action"=timerAction_typdef."Start Timer") -> ()  [unwired: 9 in, 1 out]
              }
              frame True {
                # "when to is true\nand"
                n448 = case shown="False" w1206 {
                  tunnel: w1207 -> [w1213 _]
                  tunnel: [w1211 w1226] -> w1208
                  tunnel: w1205 -> [w1209 w1227]
                  frame False {
                    n449 = call "FindControlByName_VEPS.vi"("control name"="Op Out", "vi refnum"=w1213) -> ("control refnum"=w1215:refnum<vi>)  [unwired: 2 in, 1 out]
                    n450 = property class="Ctl"(reference=w1215) -> ("Value"=w1214:variant)  [unwired: 1 in, 2 out]
                    n451 = Variant To Data(type=op_typdef."Idle" ("Op Out"), Variant=w1214) -> (data=w1212:T24)  [unwired: 1 in, 1 out]
                    n452 = case shown="\"Idle\", Default" w1212 {
                      tunnel: [w1217 "Main: Check Chamber Pressure" "Idle\nMacro: Exit"] -> w1211
                      tunnel: w1209 -> [w1218 _ _]
                      frame "Idle", Default {
                        n453 = call "MID-VAC Timer.vi"("TO sec (Start timer)"=30.0, "Action"=timerAction_typdef."Start Timer") -> ()  [unwired: 9 in, 1 out]
                        n454 = Concatenate Strings("Main: Check GPM GVM Mode Status>>", w1218) -> (w1217:string)
                      }
                      frame "Continue to Wait" {
                        # "Continue to wait. Reset Timer"
                        n455 = call "MID-VAC Timer.vi"("TO sec (Start timer)"=30.0, "Action"=timerAction_typdef."Start Timer") -> ()  [unwired: 9 in, 1 out]
                      }
                      frame "Exit" {
                      }
                    }
                  }
                  frame True {
                    n456 = Concatenate Strings("Main: Check GPM GVM Mode Status>>", w1227) -> (w1226:string)
                  }
                }
              }
            }
          }
        }
        n457 = call "Generate User Event.vi"("Add(t)/Remove(f) Event"=w1128, "error in (no error)"=w1137, "User Event in"=w1138, "Status Array In"=w1140, "Error Codes"=w1139) -> ("error out"=w1136:errorcluster)  [unwired: 5 in, 1 out]
        n458 = call "MID-VAC Timer.vi"("Action"=timerAction_typdef."Timer Running") -> ("TO"=w1132:bool)  [unwired: 10 in]
        n459 = And(x=w1128, y=w1132) -> (x .and. y?=w1131:bool)
        n460 = call "Generate TO event.vi"("Boolean"=w1131, "message"="GPM or GVM Modes are still ON.\nClick Continue to wait for another 30 seconds.\nClick on Exit to QUIT", "User Event in"=w1129) -> ()  [unwired: 9 in]
        n461 = call <vilib>:"Add State(s) to Queue__jki_lib_state_machine.vi"("State(s) in Front (\"\")"=w1126, "State(s) in (\"\")"=w1143) -> ("States Out"=w1142:string)  [unwired: 13 in]
      }
      frame "Main: Check Turbo Gate Valves" {
        w1240 = Error_codes."002-Turbo gate valve status" ("Error Codes")
        w1246 = T32[] [enum."Is M123 Turbo Gate Valve Closed?", enum."Is OAP Turbo Gate Valve Closed?", enum."Is BTL Turbo Gate Valve Closed?", enum."Is TARGET1 Turbo Gate Valve Closed?", enum."Is TAREGT2 Turbo Gate Valve Closed?", enum."Is BTL2 Turbo Gate Valve Closed?", enum."Is HPD Turbo Gate Valve Closed?"] items=["No Action", "Is EC GPM Mode ON?", "Is EC GPM Mode Off?", "Is EC GVM Mode ON?", "Is EC GVM Off?", "Is  EC GPM or GVM Mode ON?", "Is LB GPM Mode ON?", "Is LB GPM Mode Off?", "Is LB GVM Mode ON?", "Is LB GVM Mode Off?", "Is  LB GPM or GVM Mode ON?", "Is M123 Turbo Gate Valve Opened? ", "Is M123 Turbo Gate Valve Closed?", "Is OAP Turbo Gate Valve Opened?", "Is OAP Turbo Gate Valve Closed?", "Is BTLTurbo Gate Valve Opened?", "Is BTL Turbo Gate Valve Closed?", "Is TARGET Turbo Gate Valve 1Opened?", "Is TARGET1 Turbo Gate Valve Closed?", "Is TARGET Turbo Gate Valve 2 Opened?", "Is TAREGT2 Turbo Gate Valve Closed?", "Is BTL2 Turbo Gate Valve Opened?", "Is BTL2 Turbo Gate Valve Closed?", "Is HPD Turbo Gate Valve Opened?", "Is HPD Turbo Gate Valve Closed?", "Is COMP to M123 gate Valve Opened?", "Is COMP to M123 Valve Closed?", "Is HPBD Gate Valve Opened?", "Is HPBD Gate Valve Closed?", "Is M123 to OAP gate valve opened?", "Is M123 to OAP gate valve closed?", "Is OAP to BLT gate valve opened?", "Is OAP to BTL Gate Valve Closed?", "Is BLT to TARGET gate valve opened?", "Is BTL to TARGET Gate Valve Closed?", "Is TARGET to BLT2 gate valve opened?", "Is TARGET to BTL2 Gate Valve Closed?", "Is BLT2 to HPD gate valve opened?", "Is BTL2 to HPD Gate Valve Closed?", "Is COMP at Atmospheric Pressure?", "Is M123 at Atmospheric Pressure?", "Is BeamDump at Atmospheric Pressure?", "Is OAP at Atmospheric Pressure?", "Is BLT at Atmospheric Pressure", "Is TARGET at Atmospheric Pressure?", "Is BLT2 at Atmospheric Pressure?", "Is HPD at Atmospheric Pressure?", "Is the EC Roughing Pump ON?", "Is the EC Roughing Pump OFF?", "Does the EC Roughing Pump have a fault?", "Is the LB Roughing Pump ON?", "Is the LB Roughing Pump Off?", "Does the LB Roughing Pump have a fault?", "Is the EC Backing Pump ON?", "Is the EC Backing Pump OFF?", "Is the LB Backing Pump ON?", "Is the LB Backing Pump OFF?", "Does the EC Backing Pump have a fault?", "Does the LB Backing Pump have a fault?", "Is the EC Backing Pipe at Atmospheric Pressure", "Is the LB Backing Pipe at Atmospheric Pressure", "Is the EC Backing Manifold at Atmospheric Pressure", "s the LB Backing Manifold at Atmospheric Pressure?", "Is the EC Roughing Pipe at Atmospheric Pressure", "Is the LB Roughing Pipe at Atmospheric Pressure?", "Is the EC Roughing Manifold at Atmospheric Pressure", "Is the LB Roughing Manifold at Atmospheric Pressure", "Is LB Backing Manifold Valve Opened?", "Is EC Backing Manifold Valve Opened?", "Is LB Roughing Manifold Valve Opened?", "Is EC Roughing Manifold Valve Opened?", "Is COMP Roughing Valve Opened?", "Is M123 Roughing Valve Opened?", "Is M123 Roughing Valve Closed?", "Is OAP Roughing Valve Opened?", "Is OAP Roughing Valve Closed?", "Is HPBD Roughing Valve Opened?", "Is HPBD Roughing Valve Closed?", "Is BTL Roughing Valve Opened?", "Is BTL Roughing Valve Closed?", "Is TARGET Roughing Valve Opened?", "Is TARGET Roughing Valve Closed?", "Is BTL2 Roughing Valve Opened?", "Is BTL2 Roughing Valve Closed?", "Is HPD Roughing Valve Opened?", "Is HPD Roughing Valve Closed?", "Is COMP Turbo Backing Valve Opened?", "Is M123 Turbo Backing Valve Opened", "Is HPBD Turbo Backing Valve Opened?", "Is OAP Turbo Backing Valve Opened?", "Is BTL Turbo Backing Valve Opened?", "Is TARGET1 Turbo Backing Valve Opened?", "Is TARGET2 Turbo Backing Valve Opened?", "Is BTL2 Turbo Backing Valve Opened?", "Is HPD Turbo Backing Valve Opened?", "Is M123 Backing at MID-VAC?", "Is OAP Backing at MID-VAC?", "Is TARGET1 Backing at MID-VAC?", "Is TARGET2 Backing at MID-VAC?", "Is BTL Backing at MID-VAC?", "Is BTL2 Backing at MID-VAC?", "Is HPD Backing at MID-VAC?", "Is M123 Turbo in Normal Operation", "Is COMP Turbo in Normal Operation", "Is OAP Turbo in Normal Operation", "Is BTL Turbo in Normal Operation", "Is TARGET1 Turbo in Normal Operation", "Is TARGET2 Turbo in Normal Operation", "Is BTL2 Turbo in Normal Operation", "Is HPD Turbo in Normal Operation", "Is M123 at MID-VAC?", "Is OAP at MID-VAC?", "Is COMP at MID-VAC?", "Is BTL at MID-VAC?", "Is TARGET at MID-VAC?", "Is BTL2 at MID-VAC?", "Is HPD at MID-VAC?"]
        # "Interlock wants all closed."
        # "If F, then all chambers are at ATM"
        # "Event TAG"
        # "Check Conditions"
        # "Are any of the Turbo gate valves open?"
        n462 = call "GetAction.vi"("Check Condition"=w1240, "Query Array"=w1246, "input cluster"=w1231, "error in (no error)"=w1245) -> ("Status Array Out"=w1241:string[], "Generate Event?"=w1232:bool, "error out"=w1244:errorcluster)  [unwired: 6 in, 3 out]
        n463 = call "Generate User Event.vi"("Add(t)/Remove(f) Event"=w1232, "error in (no error)"=w1244, "User Event in"=w1242, "Status Array In"=w1241, "Error Codes"=w1240) -> ("error out"=w1243:errorcluster)  [unwired: 5 in, 1 out]
        n464 = Unbundle By Name(w1231) -> ("VI Refnum"=w1234:refnum<vi>)
        n465 = Not A Number/Path/Refnum?(number/path/refnum=w1234) -> (NaN/Path/Refnum?=w1233:bool)
        n466 = case shown="False" w1232 {
          tunnel: ["Main: Init State Sanity Check Array" w1262] -> w1230
          tunnel: w1234 -> [w1252 w1261]
          tunnel: w1233 -> [w1253 w1260]
          frame False {
            n467 = case shown="True" w1253 {
              tunnel: w1252 -> [_ w1256]
              frame False {
              }
              frame True {
                n468 = invoke class="VI" method="Abort VI"(reference=w1256) -> (reference out=w1254:refnum<vi>, error out=w1255:errorcluster)  [unwired: 2 in, 1 out]
                n469 = case shown="No Error" w1255 {
                  selector: w1255 -> [w1258 _]
                  tunnel: w1254 -> [w1259 _]
                  frame No Error {
                    n470 = Close Reference(reference=w1259, error in (no error)=w1258) -> (error out=w1257:errorcluster)
                    n471 = invoke on="User Input Panel" class="SubPnl" method="Remove VI"(error in=w1257) -> ()  [unwired: 2 in, 3 out]
                  }
                  frame Error {
                  }
                }
              }
            }
            n472 = call "MID-VAC Timer.vi"("TO sec (Start timer)"=20.0, "Action"=timerAction_typdef."Start Timer") -> ()  [unwired: 9 in, 1 out]
          }
          frame True {
            # "when to is true\nand"
            n473 = case shown="False" w1260 {
              tunnel: w1261 -> [w1266 _]
              tunnel: [w1264 "Main: Check COMP gate valve"] -> w1262
              frame False {
                n474 = call "FindControlByName_VEPS.vi"("control name"="Op Out", "vi refnum"=w1266) -> ("control refnum"=w1268:refnum<vi>)  [unwired: 2 in, 1 out]
                n475 = property class="Ctl"(reference=w1268) -> ("Value"=w1267:variant)  [unwired: 1 in, 2 out]
                n476 = Variant To Data(type=op_typdef."Idle" ("Op Out"), Variant=w1267) -> (data=w1265:T24)  [unwired: 1 in, 1 out]
                n477 = case shown="\"Idle\", Default" w1265 {
                  tunnel: ["Main: Check COMP gate valve" "Main: Check COMP gate valve" "Idle\nMacro: Exit"] -> w1264
                  frame "Idle", Default {
                    n478 = call "MID-VAC Timer.vi"("TO sec (Start timer)"=30.0, "Action"=timerAction_typdef."Start Timer") -> ()  [unwired: 9 in, 1 out]
                  }
                  frame "Continue to Wait" {
                    # "Continue to wait. Reset Timer"
                    n479 = call "MID-VAC Timer.vi"("TO sec (Start timer)"=30.0, "Action"=timerAction_typdef."Start Timer") -> ()  [unwired: 9 in, 1 out]
                  }
                  frame "Exit" {
                  }
                }
              }
              frame True {
              }
            }
          }
        }
        n480 = call "MID-VAC Timer.vi"("Action"=timerAction_typdef."Timer Running") -> ("TO"=w1238:bool)  [unwired: 10 in]
        n481 = And(x=w1232, y=w1238) -> (x .and. y?=w1237:bool)
        n482 = call "Generate TO event.vi"("Boolean"=w1237, "message"="Some of the turbo valves are open.\nIgnore and continue (interlock will shut the Turbo Gate Valves.)\nStop and Exit.(Restart the Pump down after all turbo valves have been manually closed)", "User Event in"=w1235) -> ()  [unwired: 9 in]
        n483 = call <vilib>:"Add State(s) to Queue__jki_lib_state_machine.vi"("State(s) in (\"\")"=w1248, "State(s) at Back (\"\")"=w1230) -> ("States Out"=w1247:string)  [unwired: 13 in]
      }
      frame "Main: Init State Sanity Check Array" {
